vi "Add Abyss Lines to Grid.vi"(11 "Grig in":T1[][](array[typedef])) -> (3 "Array":T1[][](array[typedef]))   [LabVIEW 2020]
uses:
  RB ENUM_Space ID.ctl
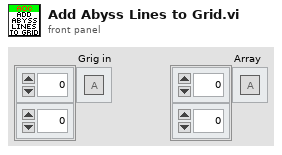
[diagram p1: front panel]
types:
  T1 = typedef "RB ENUM_Space ID.ctl" = enum32{"Air", "Sand", "Rock", "Start", "Abyss"}
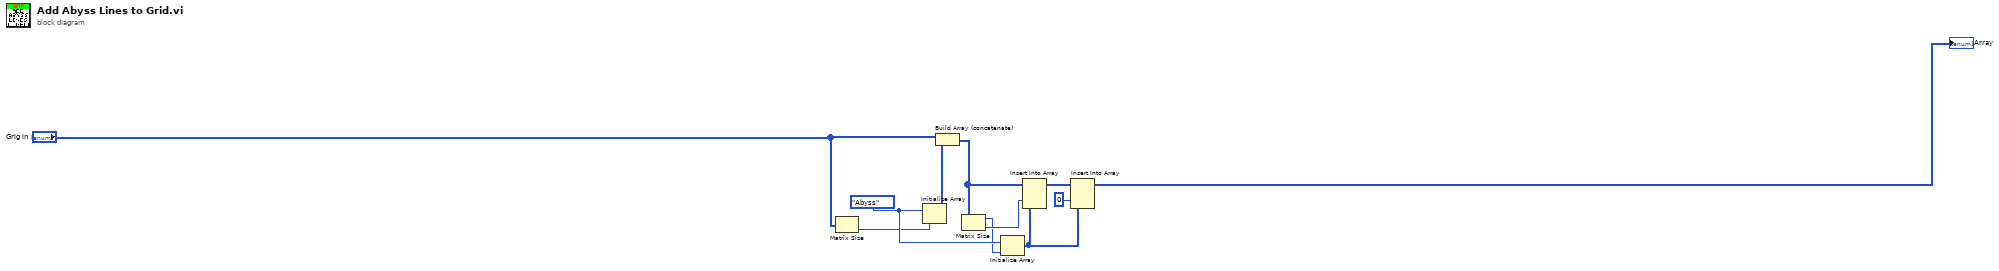
[diagram p0: block diagram]
diagram:
  w6 = RB_ENUM_Space_ID."Abyss" ("Space")
  n1 = Matrix Size(0:"Grig in") -> (2:w1:i32)  [unwired: 1 out]
  n2 = Initialize Array(w6, w1) -> (w2:T1[])
  n3 = Build Array (concatenate)("Grig in", w2) -> (w4:T1[][])
  n4 = Matrix Size(0:w4) -> (1:w5:i32, 2:w8:i32)
  n5 = Initialize Array(w6, w5) -> (w7:T1[])
  n6 = Insert Into Array(array=w4, index (col)=w8, new element=w7) -> (w3:T1[][])  [unwired: 1 in]
  n7 = Insert Into Array(array=w3, index (col)=0 ("disabled index (col)"), new element=w7) -> (→"Array":T1[][])  [unwired: 1 in]
